vi "kalman filter.vi"(9 "U in":T1, 10 "Y in":T1) -> (2 "X hat":T1)   [LabVIEW 2019]
uses:
  <vilib>/Analysis/NI_AALBase.lvlib
  <vilib>/Analysis/baseanly.llb/Real A x B.vi
  <vilib>/Analysis/NI_AALPro.lvlib
  <vilib>/Analysis/baseanly.llb/A x Vector.vi
  <vilib>/Analysis/Matrix/NI_Matrix.lvlib
  <vilib>/Analysis/Matrix/Numeric/Add/Add - RM,RM.vi
  <vilib>/silver_ctls/ArrayMatrixCluster/Real Matrix NI_Silver.ctl
panel:
  in  "D":T1
  in  "B":T1
  in  "C":T1
  in  "A":T1
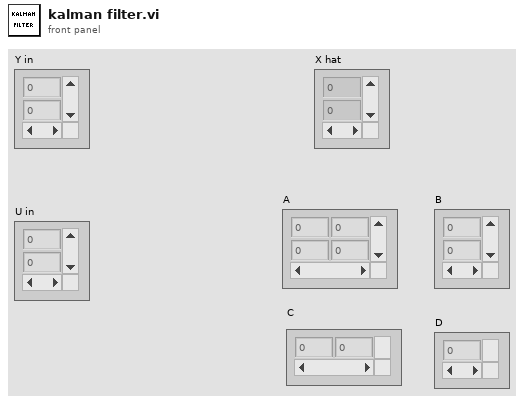
[diagram p1: front panel]
types:
  T1 = typedef "Real Matrix NI_Silver.ctl" = dbl[][]
  T2 = typedef "NI_Matrix.lvlib/RealMatrix.ctl" = dbl[][]
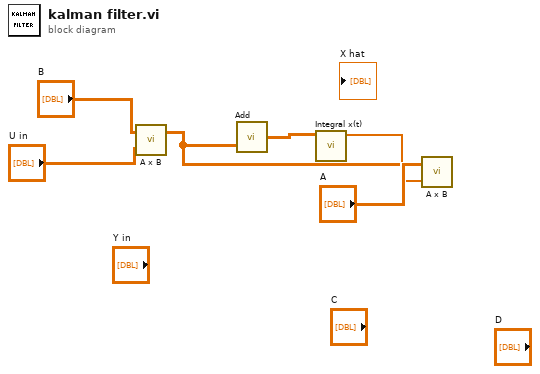
[diagram p0: block diagram]
diagram:
  n1 = call-poly <vilib>:"A x B.vi"("B"="U in", "A"="B") -> ("A x B"=w2:T2)  [unwired: 1 out]
  n2 = call-poly <vilib>:"Add.vi"("Real Matrix B"=w2) -> ("A + B"=w1:T2)  [unwired: 1 in]
  n3 = call <vilib>:"Integral x(t).vi"("X"=w1) -> ("Integral X"=w3:dbl[])  [unwired: 9 in, 1 out]
  n4 = call-poly <vilib>:"A x B.vi"("A x Vector"=w2, "Vector"=w3, "A"="A") -> ()  [unwired: 1 out]
